vi "Read Min.vi"(8 "error in (no error)":errorcluster, 11 "Online_Statistic in":refnum<class "Online_Statistic.lvclass">) -> (0 "error out":errorcluster, 2 "Min":dbl, 3 "Online_Statistic out":refnum<class "Online_Statistic.lvclass">)   [LabVIEW 2021, in "Online_Statistic.lvclass"]
uses:
  Online_Statistic.lvclass
  Online_Statistic.lvclass/Online_Statistic.ctl
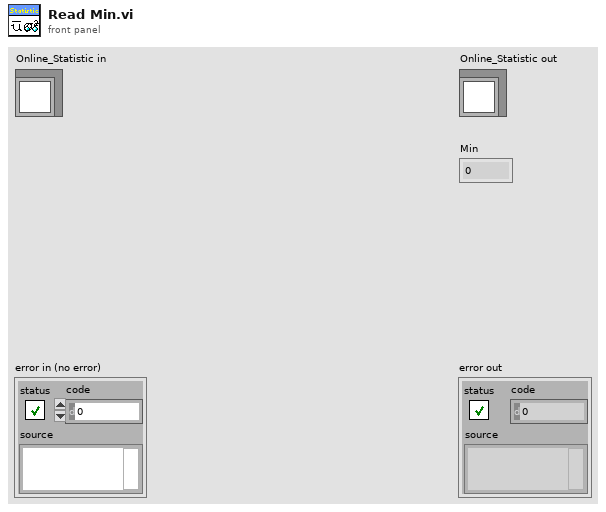
[diagram p1: front panel]
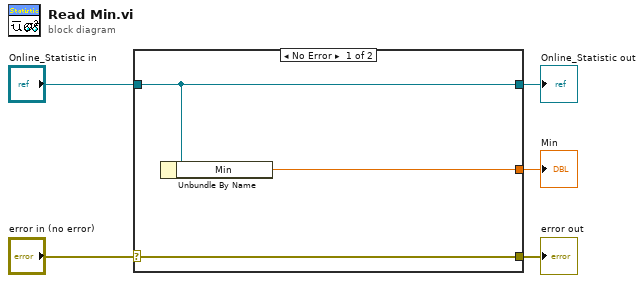
[diagram p0: block diagram]
diagram:
  n1 = case shown="No Error" "error in (no error)" {
    selector: "error in (no error)" -> [w8 w9]
    tunnel: [w8 w9] -> w4
    tunnel: [w7 w10] -> w2
    tunnel: "Online_Statistic in" -> [w7 w10]
    tunnel: [w6 _] -> w1
    frame No Error {
      n2 = Unbundle By Name(w7) -> ("Min"=w6:dbl)
    }
    frame Error {
    }
  }
  "error out" <- w4
  "Online_Statistic out" <- w2
  "Min" <- w1
